vi "Aqisicao_V3.vi"() -> ()   [LabVIEW 2020]
uses:
  MyFirmware-V3/State_Enum.ctl
  <vilib>/Platform/TimedLoop/XDataNode/timing_clust.ctl
  <vilib>/Platform/TimedLoop/XDataNode/nitl_modes.ctl
  <vilib>/Platform/TimedLoop/XDataNode/wakeup.ctl
  <vilib>/DAQmx/read.llb/DAQmx Read (Analog Wfm 1Chan NSamp).vi
  <vilib>/Analysis/baseanly.llb/Mean (DBL).vi
  <vilib>/DAQmx/configure/timing.llb/DAQmx Timing (Sample Clock).vi
  <vilib>/DAQmx/miscellaneous.llb/DAQmx Fill In Error Info.vi
  <vilib>/platform/TimedLoop/XDataNode/XDataNode.xnode
  <vilib>/Analysis/NI_AALBase.lvlib
  <vilib>/Platform/TimedLoop/XDataNode/XDNodeRunTimeDep.lvlib
panel:
  out "Numeric":i32
  in  "Suspender":bool
  in  "Menu 2":cluster{"Cancel Button 2":bool, "stop":bool}
  in  "Filename":path=path "C:/Users/jorge/SynologyDrive/ARDUINO/Projects/Filament/MyFirmware-V4/Exp_1.txt"
  in  "Write File?»":bool=TRUE
  in  "Freq. Amostragem":dbl=100.0
  out "mean":dbl=nan format="%0.4f"
  out "Waveform Graph":dbl[](graph)
  # "Hz"
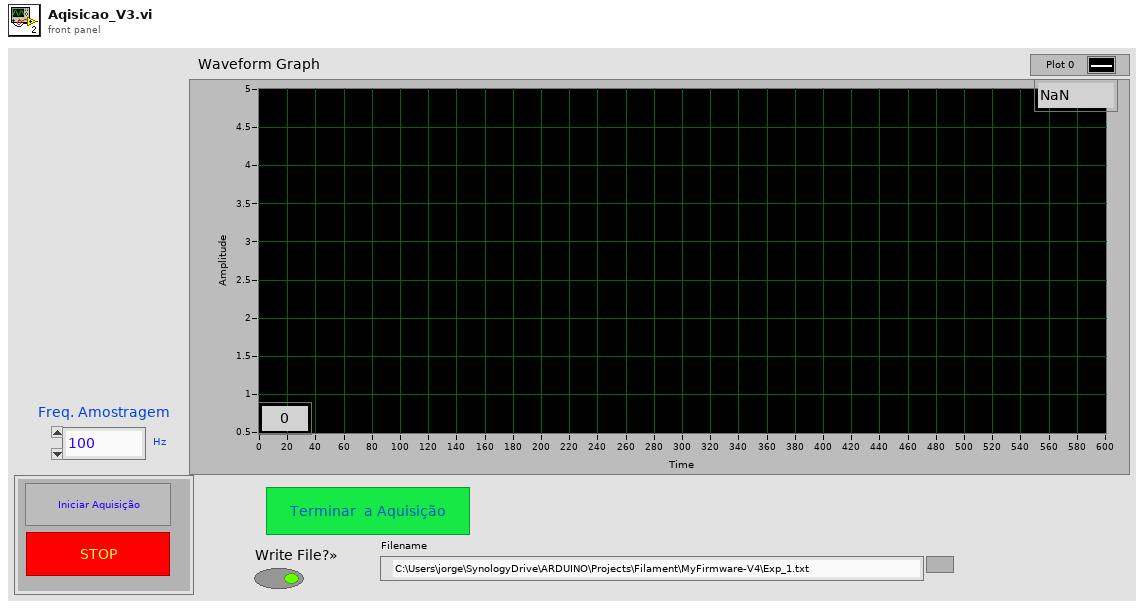
[diagram p1: front panel]
types:
  T1 = typedef "State_Enum.ctl" = enum32{"Idle", "Acquire", "Stop"}
  T2 = typedef "XDNodeRunTimeDep.lvlib/timing_clust.ctl" = cluster{"Expected End [f-1]":u64, "Actual End [f-1]":u64, "Finished Late? [f-1]":bool, "Expected End [i-1]":u64, "Actual End [i-1]":u64, "Finished Late? [i-1]":bool, "Expected Start [i]":u64, "Actual Start [i]":u64, "Expected Start [f]":u64, "Actual Start [f]":u64, "Source Name":string, "Structure Name":string, "Period":i64, "Deadline":i64, "Offset":i64, "Start":i64, "Priority":i32, "Timeout":i32, "Mode":T3, "Wakeup Reason":T4, "Error":errorcluster, "Source Type":string, "Secondary Source Type":string, "Global End Time":u64, "Global Start Time":u64, "Frame Duration":u64, "Iteration Duration":u64, "Assigned CPU":i32, "I/O Scan Engine Mode":u32}
  T3 = typedef "XDNodeRunTimeDep.lvlib/nitl_modes.ctl" = enum32{"No Change", "Process missed periods, maintain original phase", "Discard missed periods, maintain original phase", "Process missed periods, ignore original phase", "Discard missed periods, ignore original phase"}
  T4 = typedef "XDNodeRunTimeDep.lvlib/wakeup.ctl" = enum32{"Normal", "Aborted", "Asynchronous wakeup", "Timing source error", "Timed loop error", "Timeout"}
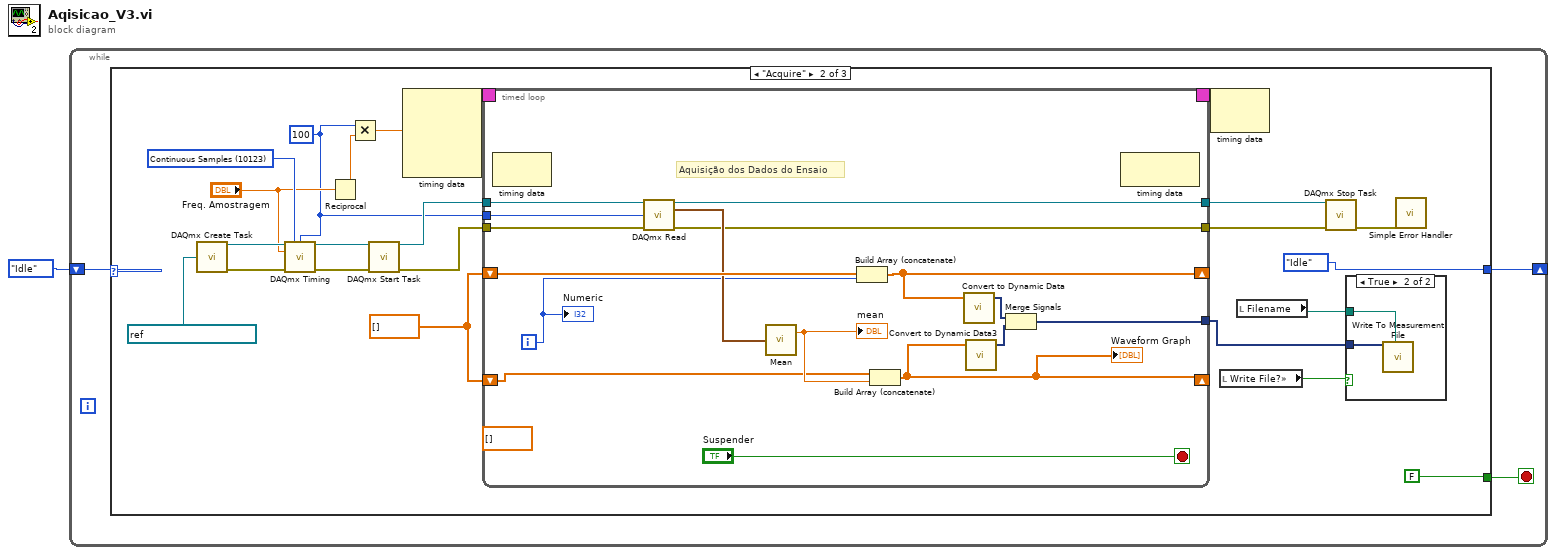
[diagram p0: block diagram]
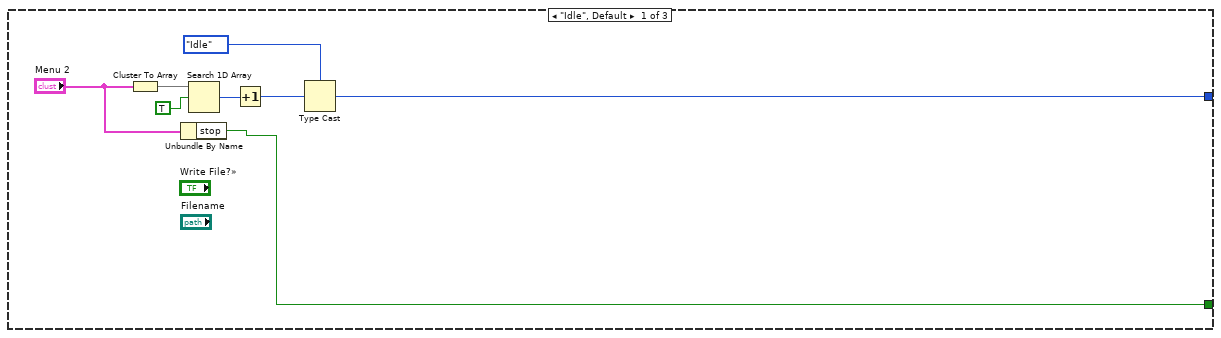
[diagram p2: hidden frame]
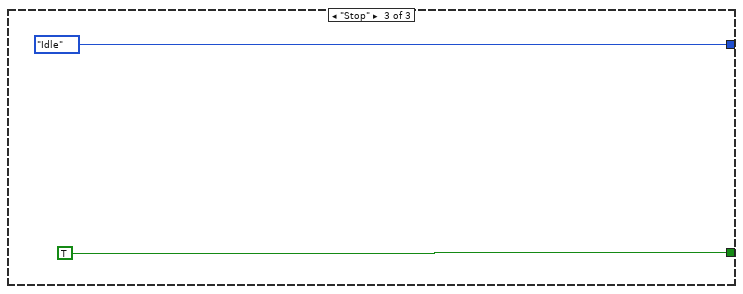
[diagram p4: hidden frame]
diagram:
  n1 = while {
    shift-right: [w4] -> _
    shift-left: State_Enum."Idle" ("State Enum") -> [w3]
    stop <- w2 stop-if-true
    n2 = case shown="\"Acquire\"" w3 {
      tunnel: [w8 State_Enum."Idle" ("State Enum") State_Enum."Idle" ("State Enum")] -> w4
      tunnel: [w5 FALSE TRUE ("stop")] -> w2
      frame "Idle", Default {
        n3 = Cluster To Array(cluster="Menu 2") -> (array=w12:bool[])
        n4 = Unbundle By Name("Menu 2") -> ("stop"=w5:bool)
        n5 = Search 1D Array(1D array=w12, element=TRUE) -> (index of element=w11:i32)  [unwired: 1 in]
        n6 = Increment(x=w11) -> (x+1=w10:i32)
        n7 = Type Cast(type=State_Enum."Idle" ("State Enum"), x=w10) -> (*(type *) &x=w8:T1)
      }
      frame "Acquire" {
        w13 = 100 ("samples per channel")
        w23 = 10123 items=["Finite Samples"=10178, "Continuous Samples"=10123, "Hardware Timed Single Point"=12522] ("sample mode")
        w32 = dbl[] []
        (unwired) dbl[] []
        n8 = call <vilib>:"DAQmx Create Task.vi"("global virtual channels"=refnum<k21> "MyVoltageChannel") -> ("task out"=w29:refnum<k21>, "error out"=w28:errorcluster)  [unwired: 13 in]
        n9 = call-poly <vilib>:"DAQmx Timing.vi"("task/channels in"=w29, "sample mode"=w23, "samples per channel"=w13, "rate"="Freq. Amostragem", "error in"=w28) -> ("task out"=w26:refnum<k21>, "error out"=w27:errorcluster)  [unwired: 9 in]
        n10 = Reciprocal(x="Freq. Amostragem") -> (1/x=w15:dbl)
        n11 = Multiply(x=w13, y=w15) -> (x*y=w14:dbl)
        n12 = call <vilib>:"DAQmx Start Task.vi"("task/channels in"=w26, "error in"=w27) -> ("task out"=w25:refnum<k21>, "error out"=w24:errorcluster)  [unwired: 12 in]
        n13 = node-c288(w14) -> (w18:T2)  [unwired: 3 in]
        n14 = timed-loop {
          shift-right: [w36] -> _
          shift-left: w32 -> [w48]
          shift-right: [w37] -> _
          shift-left: w32 -> [w47]
          tunnel: [w39] -> w33
          tunnel: w25 -> [w45]
          tunnel: w24 -> [w44]
          tunnel: w13 -> [w43]
          tunnel: [w41] -> w22
          tunnel: [w40] -> w21
          timing: w18 -> [_]
          timing-out: [_] -> w17
          i -> [w38]
          stop <- "Suspender" stop-if-true
          # "Aquisição dos Dados do Ensaio"
          n15 = node-c288() -> ()  [unwired: 1 in, 1 out]
          n16 = call-poly <vilib>:"DAQmx Read.vi"("task/channels in"=w45, "number of samples per channel"=w43, "error in"=w44) -> ("task out"=w41:refnum<k21>, "data"=w42:waveform(dbl), "error out"=w40:errorcluster)  [unwired: 10 in]
          n17 = call-poly <vilib>:"Mean.vi"("X"=w42) -> ("mean"=w51:dbl)  [unwired: 1 out]
          "mean" <- w51
          n18 = Build Array (concatenate)(w48, w38) -> (w36:dbl[])
          n19 = Build Array (concatenate)(w47, w51) -> (w37:dbl[])
          "Waveform Graph" <- w37
          n20 = call "Convert to Dynamic Data"("Array"=w36) -> ("Dynamic Data Type"=w50:dynamicdata)  [unwired: 3 in]
          n21 = call "Convert to Dynamic Data3"("Array"=w37) -> ("Dynamic Data Type"=w49:dynamicdata)  [unwired: 3 in]
          n22 = Merge Signals(w50, w49) -> (w39:dynamicdata)
          n23 = node-c288() -> ()  [unwired: 1 in, 1 out]
          "Numeric" <- w38
        }
        n24 = node-c288(w17) -> ()  [unwired: 1 out]
        n25 = local read "Write File?»"() -> (w31:bool)
        n26 = local read "Filename"() -> (w30:path)
        n27 = call <vilib>:"DAQmx Stop Task.vi"("task/channels in"=w22, "error in"=w21) -> ("error out"=w20:errorcluster)  [unwired: 12 in, 1 out]
        n28 = case shown="True" w31 {
          tunnel: w33 -> [_ w59]
          tunnel: w30 -> [_ w58]
          frame False {
          }
          frame True {
            n29 = call "Write To Measurement File"("Signals"=w59, "Filename"=w58) -> ()  [unwired: 15 in, 3 out]
          }
        }
        n30 = call <vilib>:"Simple Error Handler.vi"("error in (no error)"=w20) -> ()  [unwired: 4 in, 5 out]
      }
      frame "Stop" {
      }
    }
  }
